vi "Had_acquisition_started.vi"(7 "error in (no error)":errorcluster, 10 ".NET Refnum in":refnum<k24>) -> (0 "error out":errorcluster, 2 "bValue":bool, 3 ".NET Refnum out":refnum<k24>)   [LabVIEW 2021]
uses:
  C:/Program Files/Thorlabs/Scientific Imaging/ThorCam/uc480DotNet.dll
  Program Files/Thorlabs/Scientific Imaging/ThorCam/uc480DotNet.dll
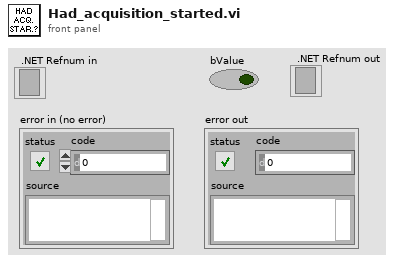
[diagram p1: front panel]
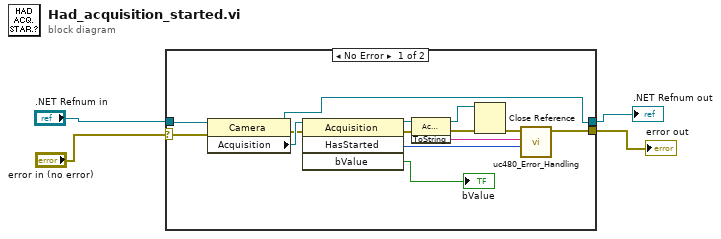
[diagram p0: block diagram]
diagram:
  n1 = case shown="No Error" "error in (no error)" {
    selector: "error in (no error)" -> [w6 w19]
    tunnel: ".NET Refnum in" -> [w18 w20]
    tunnel: [w14 w19] -> w3
    tunnel: [w5 w20] -> w1
    frame No Error {
      n2 = property class="Camera"(reference=w18, error in=w6) -> (reference out=w5:refnum<k24>, error out=w7:errorcluster, "Acquisition"=w8:refnum<k24>)
      n3 = invoke class="Acquisition" method="HasStarted"(reference=w8, error in=w7) -> (reference out=w10:refnum<k24>, error out=w11:errorcluster, "HasStarted"=w12:i32, "bValue"=→"bValue":bool)  [unwired: 2 in]
      n4 = invoke class="Acquisition" method="ToString"(reference=w10, error in=w11) -> (reference out=w17:refnum<k24>, error out=w15:errorcluster, "ToString"=w9:string)  [unwired: 1 in]
      n5 = Close Reference(reference=w17, error in (no error)=w15) -> (error out=w16:errorcluster)
      n6 = call "uc480_Error_Handling.vi"("Error Code"=w12, "Error String"=w9, "Error In"=w16) -> ("Error Out"=w14:errorcluster)  [unwired: 8 in]
    }
    frame Error {
    }
  }
  "error out" <- w3
  ".NET Refnum out" <- w1
